vi "读取数据库.vi"(5 "精度(6)":i16=2, 7 "condition":string, 8 "error in (no error)":errorcluster caption="错误输入（无错误）", 9 "database":string="database1.mdb", 10 "显示项":string[](array[string]), 11 "组合框":string(combo)) -> (0 "error out":errorcluster caption="错误输出", 1 "columns":string[](array[string]), 2 "data":variant[][](array[variant]), 3 "表格":string[][](table))   [LabVIEW 2016]
uses:
  <vilib>/Utility/sysdir.llb/System Directory Type.ctl
  <vilib>/addons/database/Connection.llb/DB Tools Open Connec (String).vi
  <vilib>/addons/database/_DB Variant To Data/Database Variant To Data.xnode
  <vilib>/addons/database/NI_Database_API.lvlib
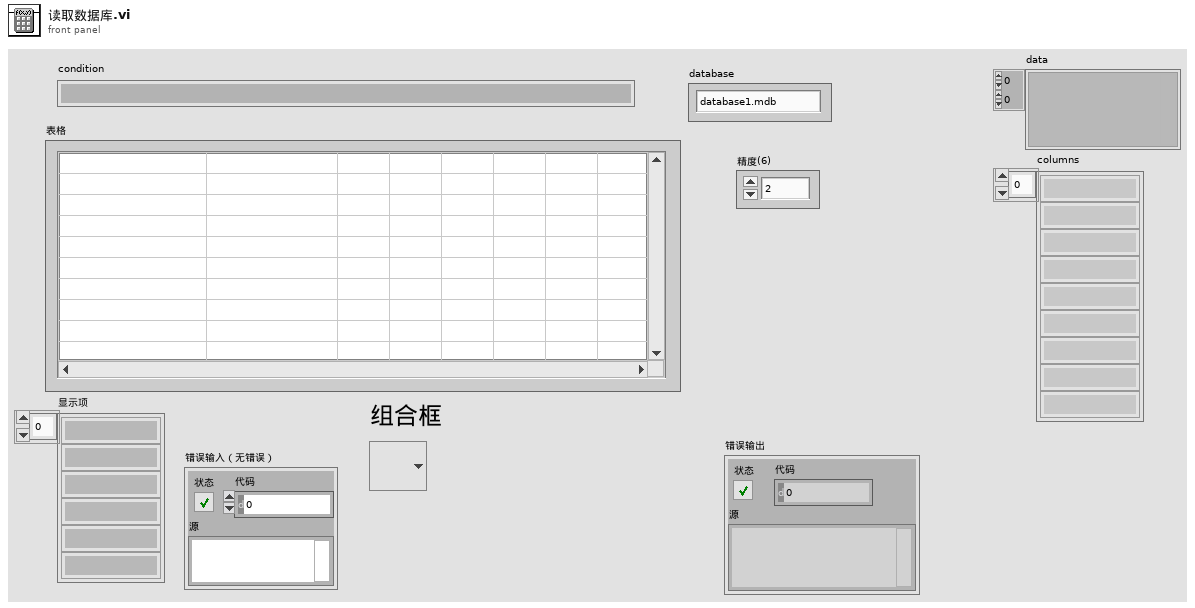
[diagram p1: front panel]
types:
  T1 = typedef "System Directory Type.ctl" = i32
  T2 = typedef "NI_Database_API.lvlib/Conn ObjectReference.ctl" = refnum<k1>
  T3 = typedef "NI_Database_API.lvlib/DB Tools DataTypes.ctl" = enum16{"String", "Long (I32)", "Single (SGL)", "Double (DBL)", "Date/Time", "Binary"}
  T4 = cluster{"name":string, "database data type":T3, "defined size":i32}[]
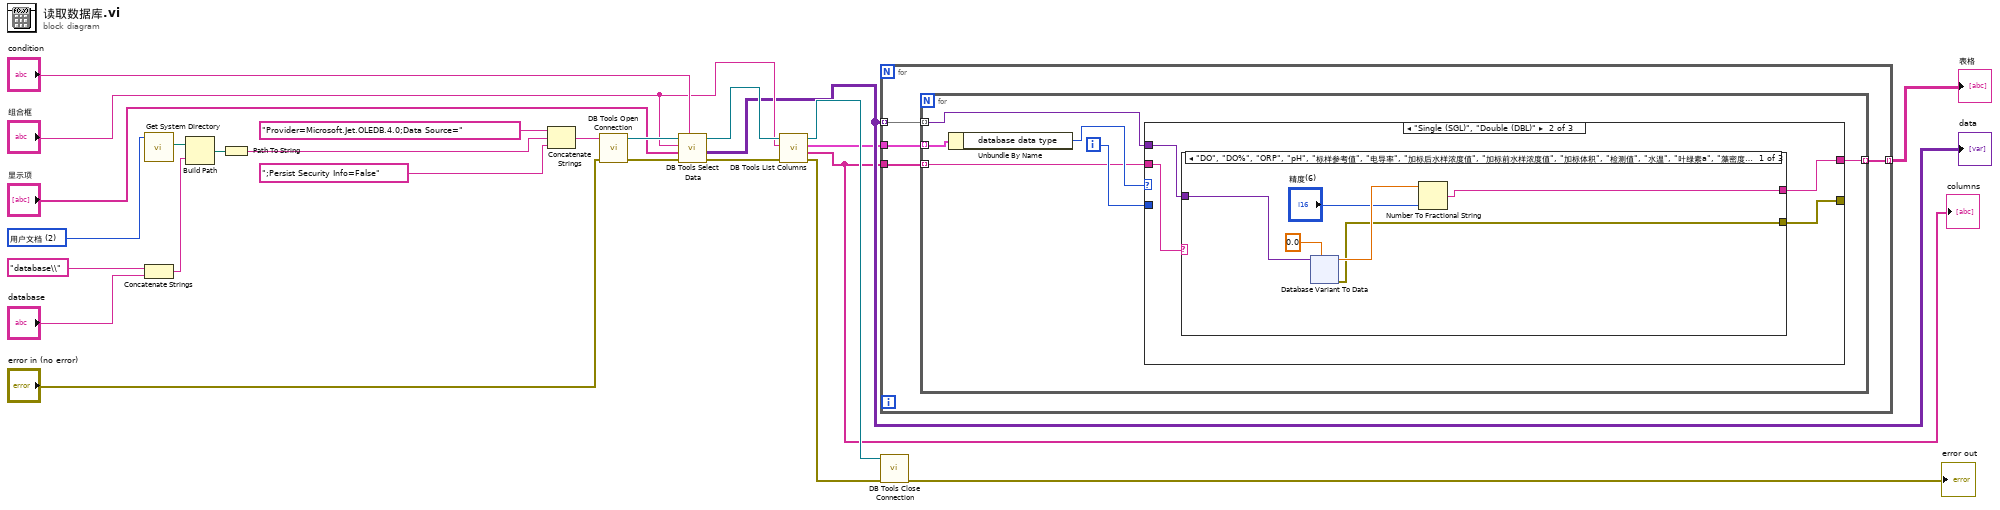
[diagram p0: block diagram]
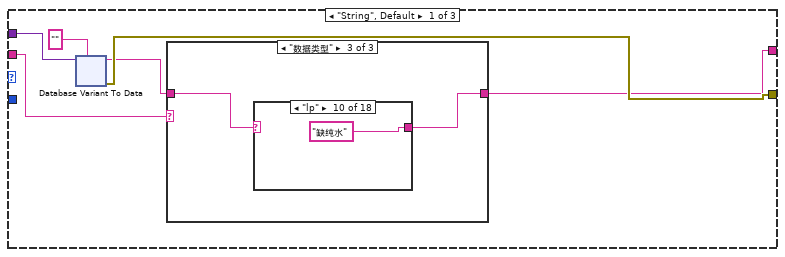
[diagram p2: hidden frame]
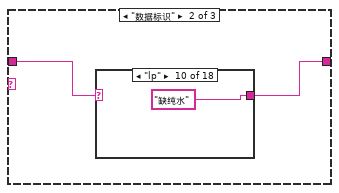
[diagram p4: hidden frame]
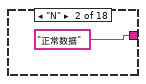
[diagram p6: hidden frame]
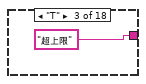
[diagram p7: hidden frame]
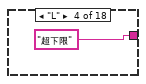
[diagram p8: hidden frame]
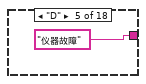
[diagram p9: hidden frame]
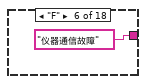
[diagram p10: hidden frame]
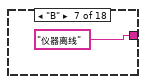
[diagram p11: hidden frame]
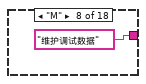
[diagram p12: hidden frame]
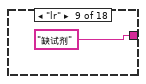
[diagram p13: hidden frame]
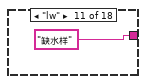
[diagram p14: hidden frame]
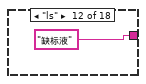
[diagram p15: hidden frame]
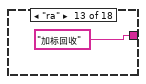
[diagram p16: hidden frame]
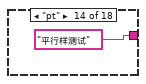
[diagram p17: hidden frame]
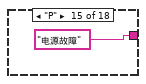
[diagram p18: hidden frame]
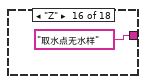
[diagram p19: hidden frame]
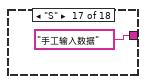
[diagram p20: hidden frame]
diagram:
  w11 = T1 2 items=["用户目录"=0, "用户桌面"=1, "用户文档"=2, "用户应用程序数据"=3, "用户设置"=4, "用户临时目录"=5, "公共文档"=6, "公共应用程序数据"=7, "公共设置"=8, "公共缓存"=13, "系统核心库"=9, "系统安装库"=10, "应用程序文件"=11, "启动盘根目录"=12] ("system directory type")
  n1 = call <vilib>:"Get System Directory.vi"("system directory type"=w11) -> ("system directory"=w10:path)  [unwired: 10 in]
  n2 = Concatenate Strings("database\\" ("名称或相对路径"), "database") -> (w7:string)
  n3 = Build Path(base path=w10, name or relative path=w7) -> (appended path=w12:path)
  n4 = Path To String(path=w12) -> (string=w13:string)
  n5 = Concatenate Strings("Provider=Microsoft.Jet.OLEDB.4.0;Data Source=", w13, ";Persist Security Info=False") -> (w9:string)
  n6 = call-poly <vilib>:"DB Tools Open Connection.vi"("error in (no error)"="error in (no error)", "connection information"=w9) -> ("error out"=w24:errorcluster, "connection reference"=w25:T2)  [unwired: 6 in]
  n7 = call <vilib>:"DB Tools Select Data.vi"("condition"="condition", "error in (no error)"=w24, "columns"="显示项", "table"="组合框", "connection reference"=w25) -> ("error out"=w23:errorcluster, "data"=w4:variant[][], "connection reference out"=w20:T2)  [unwired: 1 in]
  "data" <- w4
  n8 = call <vilib>:"DB Tools List Columns.vi"("error in (no error)"=w23, "table"="组合框", "connection reference"=w20) -> ("error out"=w16:errorcluster, "columns"=w1:string[], "column information"=w3:T4, "connection reference out"=w17:T2)  [unwired: 1 in]
  "columns" <- w1
  n9 = for {
    tunnel: w4 -> [w29] mode=indexing
    tunnel: w3 -> [w28]
    tunnel: [w27] -> w2 mode=indexing
    tunnel: w1 -> [w26]
    n10 = for {
      tunnel: w29 -> [w34] mode=indexing
      tunnel: w28 -> [w33] mode=indexing
      tunnel: [w31] -> w27 mode=indexing
      tunnel: w26 -> [w30] mode=indexing
      i -> [w32]
      n11 = Unbundle By Name(w33) -> ("database data type"=w35:T3)
      n12 = case shown="\"Single (SGL)\", \"Double (DBL)\"" w35 {
        tunnel: w34 -> [w41 w116 w246]
        tunnel: [w36 w117 w242] -> w31
        tunnel: w32 -> [_ _ _]
        tunnel: [w39 w118 w241] -> _
        tunnel: w30 -> [w37 w115 _]
        frame "String", Default {
          n13 = xnode "Database Variant To Data"("database variant"=w41, "type"="") -> ("data"=w38:string, "error out"=w39:errorcluster)  [unwired: 1 in]
          n14 = case shown="\"数据类型\"" w37 {
            tunnel: w38 -> [w42 w44 w64]
            tunnel: [w42 w43 w63] -> w36
            frame Default {
            }
            frame "数据标识" {
              n15 = case shown="\"lp\"" w44 {
                selector: w44 -> [w45 _ _ _ _ _ _ _ _ _ _ _ _ _ _ _ _ _]
                tunnel: [w45 "正常数据" "超上限" "超下限" "仪器故障" "仪器通信故障" "仪器离线" "维护调试数据" "缺试剂" "缺纯水" "缺水样" "缺标液" "加标回收" "平行样测试" "电源故障" "取水点无水样" "手工输入数据" "手动测试数据"] -> w43
                frame Default {
                }
                frame "N" {
                }
                frame "T" {
                }
                frame "L" {
                }
                frame "D" {
                }
                frame "F" {
                }
                frame "B" {
                }
                frame "M" {
                }
                frame "lr" {
                }
                frame "lp" {
                }
                frame "lw" {
                }
                frame "ls" {
                }
                frame "ra" {
                }
                frame "pt" {
                }
                frame "P" {
                }
                frame "Z" {
                }
                frame "S" {
                }
                frame "hd" {
                }
              }
            }
            frame "数据类型" {
              n16 = case shown="\"lp\"" w64 {
                selector: w64 -> [w65 _ _ _ _ _ _ _ _ _ _ _ _ _ _ _ _ _]
                tunnel: [w65 "正常数据" "超上限" "超下限" "仪器故障" "仪器通信故障" "仪器离线" "维护调试数据" "缺试剂" "缺纯水" "缺水样" "缺标液" "加标回收" "平行样测试" "电源故障" "取水点无水样" "手工输入数据" "手动测试数据"] -> w63
                frame Default {
                }
                frame "N" {
                }
                frame "T" {
                }
                frame "L" {
                }
                frame "D" {
                }
                frame "F" {
                }
                frame "B" {
                }
                frame "M" {
                }
                frame "lr" {
                }
                frame "lp" {
                }
                frame "lw" {
                }
                frame "ls" {
                }
                frame "ra" {
                }
                frame "pt" {
                }
                frame "P" {
                }
                frame "Z" {
                }
                frame "S" {
                }
                frame "hd" {
                }
              }
            }
          }
        }
        frame "Single (SGL)", "Double (DBL)" {
          n17 = case shown="\"DO\", \"DO%\", \"ORP\", \"pH\", \"标样参考值\", \"电导率\", \"加标后水样浓度值\", \"加标前水样浓度值\", \"加标体积\", \"检测值\", \"水温\", \"叶绿素a\", \"藻密度\"" w115 {
            selector: w115 -> [_ _ w197]
            tunnel: w116 -> [w124 w162 w200]
            tunnel: [w122 w160 w195] -> w117
            tunnel: [w120 w157 w198] -> w118
            frame "DO", "DO%", "ORP", "pH", "标样参考值", "电导率", "加标后水样浓度值", "加标前水样浓度值", "加标体积", "检测值", "水温", "叶绿素a", "藻密度" {
              n18 = xnode "Database Variant To Data"("database variant"=w124, "type"=0.0) -> ("data"=w123:dbl, "error out"=w120:errorcluster)  [unwired: 1 in]
              n19 = Number To Fractional String(number=w123, precision (6)="精度(6)") -> (F-format string=w122:string)  [unwired: 2 in]
            }
            frame "F0", "f1", "f2", "f3", "f4", "f5", "f6", "f7", "x", "信号值" {
              n20 = xnode "Database Variant To Data"("database variant"=w162, "type"=0.0) -> ("data"=w161:dbl, "error out"=w157:errorcluster)  [unwired: 1 in]
              n21 = Format Into String(format string="%#.4f" ("格式字符串"), w161) -> (resulting string=w160:string)  [unwired: 2 in, 1 out]
            }
            frame Default {
              n22 = xnode "Database Variant To Data"("database variant"=w200, "type"=0.0) -> ("data"=w196:dbl, "error out"=w198:errorcluster)  [unwired: 1 in]
              n23 = case shown="默认" w197 {
                tunnel: w196 -> [w202 w208]
                tunnel: [w201 w204] -> w195
                frame Default {
                  n24 = Format Into String(format string="%#.2f" ("格式字符串"), w202) -> (resulting string=w201:string)  [unwired: 2 in, 1 out]
                }
                frame "量程" {
                  n25 = Equal To 0?(x=w208) -> (x = 0?=w207:bool)
                  n26 = Select(t="低量程" ("格式字符串"), s=w207, f="高量程" ("格式字符串")) -> (s? t:f=w204:string)
                }
              }
            }
          }
        }
        frame "Date/Time" {
          n27 = xnode "Database Variant To Data"("database variant"=w246, "type"=timestamp(0 s since 1904-01-01) ("当前时间")) -> ("data"=w245:timestamp, "error out"=w241:errorcluster)  [unwired: 1 in]
          n28 = Format Date/Time String(time format string (%c)="%y/%m/%d %H:%M:%S" ("时间格式字符串(%c)"), seconds (now)=w245) -> (date/time string=w242:string)  [unwired: 1 in]
        }
      }
    }
  }
  "表格" <- w2
  n29 = call <vilib>:"DB Tools Close Connection.vi"("error in (no error)"=w16, "connection reference"=w17) -> ("error out"=→"error out":errorcluster)  [unwired: 5 in]
